vi "PDT Batch_v2.vi"(11 "PDT *.csv FilePath":path=path "C:/Users/dev/Downloads/PDT.csv") -> (3 "String":string)   [LabVIEW 2019]
uses:
  <vilib>/Utility/file.llb/Read Delimited Spreadsheet (string).vi
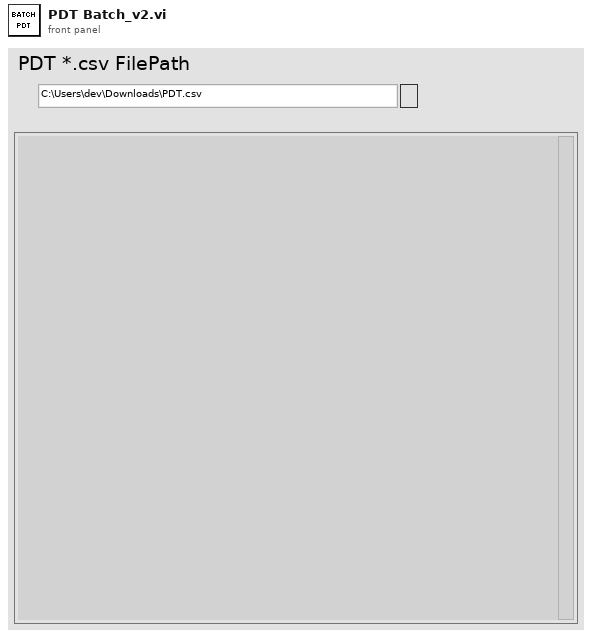
[diagram p1: front panel]
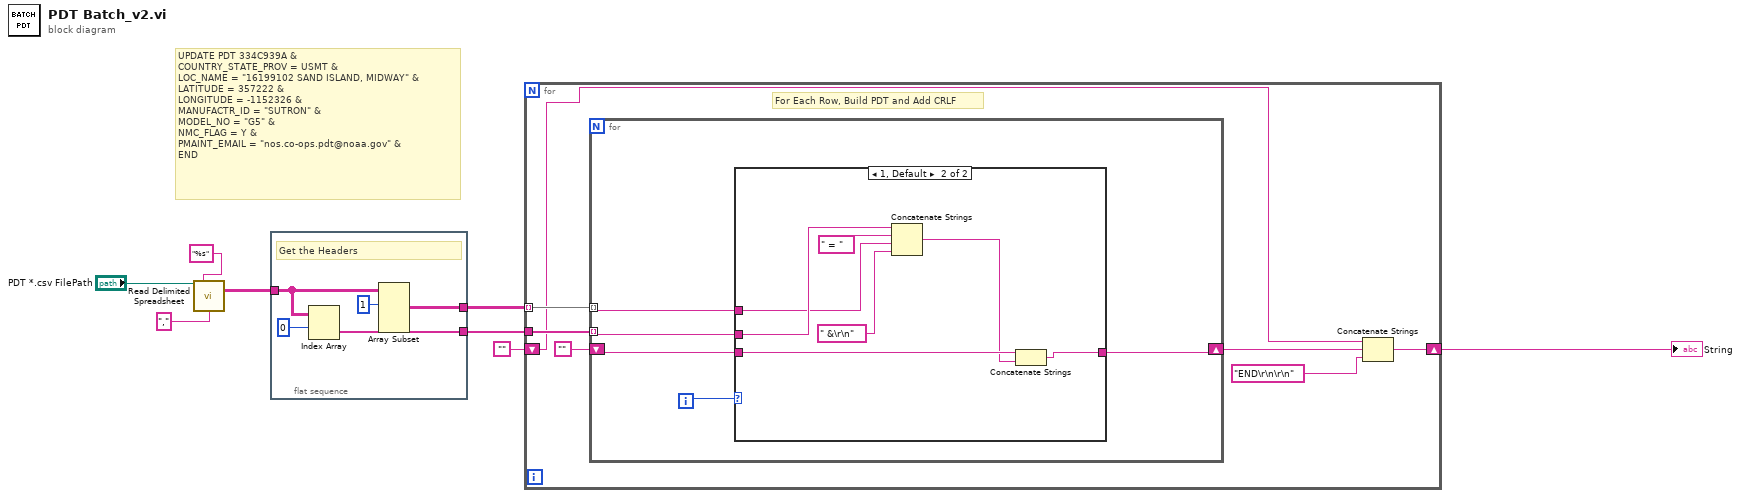
[diagram p0: block diagram]
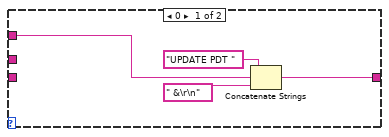
[diagram p2: hidden frame]
diagram:
  # "UPDATE PDT 334C939A &\nCOUNTRY_STATE_PROV = USMT & \nLOC_NAME = \"16199102 SAND ISLAND, MIDWAY\" & \nLATITUDE = 357222 &\nLONGITUDE = -1152326 &\nMANUFACTR_ID = \"SUTRON\" & \nMODEL_NO = \"G5\" &\nNMC_FLAG = Y &\nPMAINT_EMAIL = \"nos.co-ops.pdt@noaa.gov\" & \nEND"
  n1 = call-poly <vilib>:"Read Delimited Spreadsheet.vi"("file path (dialog if empty)"="PDT *.csv FilePath", "format (%s)"="%s" ("format (%.3f)"), "delimiter (\\t)"="," ("delimiter (\\t)")) -> ("all rows"=w5:string[][])  [unwired: 7 in, 5 out]
  n2 = flat-sequence {
    tunnel: w5 -> [w12]
    tunnel: [w11] -> w4
    tunnel: [w9] -> w3
    frame #0 {
      # "Get the Headers"
      n3 = Index Array(array=w12, index (row)=0 ("index")) -> (element=w9:string[])  [unwired: 1 in]
      n4 = Array Subset(array=w12, index (row)=1 ("index")) -> (w11:string[][])  [unwired: 3 in]
    }
  }
  n5 = for {
    tunnel: w4 -> [w20] mode=indexing
    tunnel: w3 -> [w19]
    shift-right: [w15] -> w1
    shift-left: "" -> [w17]
    # "For Each Row, Build PDT and Add CRLF"
    n6 = for {
      tunnel: w20 -> [w24] mode=indexing
      tunnel: w19 -> [w25] mode=indexing
      shift-right: [w23] -> w16
      shift-left: "" -> [w21]
      i -> [w22]
      n7 = case shown="1, Default" w22 {
        tunnel: w25 -> [_ w35]
        tunnel: w24 -> [w28 w32]
        tunnel: [w26 w34] -> w23
        tunnel: w21 -> [_ w36]
        frame 0 {
          n8 = Concatenate Strings("UPDATE PDT ", w28, " &\r\n") -> (w26:string)
        }
        frame 1, Default {
          n9 = Concatenate Strings(w35, " = " ("string"), w32, " &\r\n") -> (w30:string)
          n10 = Concatenate Strings(w36, w30) -> (w34:string)
        }
      }
    }
    n11 = Concatenate Strings(w17, w16, "END\r\n\r\n") -> (w15:string)
  }
  "String" <- w1
